vi "DecodeVireoToBotSpeak.vi"(3 "Via file":string="// Autogenerated Vireo assembly file\n// Generated on Fri Mar 27 10:48:11 2015\n\ndefine (c0 dv(.UInt32 1) )\ndefine (c1 dv(.UInt32 1) )\ndefine (c2 dv(c(\n    e(.String n0)   // Address\n    e(.String n1)   // Reply EOF\n    e(.String n2)   // Hardware\n    e(.Int8 n3)   // Retries\n    e(.Int32 n4)   // Timeout\n    e(.Boolean n5)   // Open?\n) ('' '' '' 0 0 false )) )\ndefine (c3 dv(.String '') )\n//---------------------------------------------------\n//VI Definition: BotSpeak_DIOWrite.vi\ndefine (videf1 dv(.VirtualInstrument (\n    c(\n        i(dv(.UInt32 1) local2)   // State\n        o(dv(.String '') local5)   // response\n        i(dv(c(\n            e(.String n0)   // Address\n            e(.String n1)   // Reply EOF\n            e(.String n2)   // Hardware\n            e(.Int8 n3)   // Retries\n            e(.Int32 n4)   // Timeout\n            e(.Boolean n5)   // Open?\n        ) ('' '' '' 0 0 false )) local1)   // Bot Settings\n        i(dv(.UInt32 0) local3)   // DIO Line\n        o(dv(c(\n            e(.String n0)   // Address\n            e(.String n1)   // Reply EOF\n            e(.String n2)   // Hardware\n            e(.Int8 n3)   // Retries\n            e(.Int32 n4)   // Timeout\n            e(.Boolean n5)   // Open?\n        ) ('' '' '' 0 0 false )) local4)   // Bot Settings\n    )\n    c(\n    )\n        clump(1\n        Copy(c2 local4 )\n        Copy(c3 local5 )\n//--- end of vi\n    )\n)))\n//---------------------------------------------------\n//VI Definition: TestingVI.vi\ndefine (videf2 dv(.VirtualInstrument (\n    c(\n    )\n        clump(1\n        videf1(c0 * * c1 *)\n//--- end of vi\n    )\n)))\nenqueue (videf2)\n") -> (1 "BotSpeak":string="SET DIO[1],1\n")   [LabVIEW 2012]
panel:
  out "params":T1(array[cluster])
  out "Array 3":string[](array[string])=["", "", "", "", "BotSpeak_DIOWrite.vi", "TestingVI.vi", ""]
  out "Array":T2(array[cluster])=[{"command"="define", "Contents"="c0 dv(.UInt32 1)", "previous comment"="// Generated on Fri Mar 27 10:48:11 2015"}, {"command"="define", "Contents"="c1 dv(.UInt32 1)", "previous comment"=""}, {"command"="define", "Contents"="c2 dv(c(\n    e(.String n0)   // Address\n    e(.String n1)   // Reply EOF\n    e(.String n2)   // Hardware\n    e(.Int8 n3)   // Retries\n    e(.Int32 n4)   // Timeout\n    e(.Boolean n5)   // Open?\n) ('' '' '' 0 0 false ))", "previous comment"=""}, {"command"="define", "Contents"="c3 dv(.String '')", "previous comment"=""}, {"command"="define", "Contents"="videf1 dv(.VirtualInstrument (\n    c(\n        i(dv(.UInt32 1) local2)   // State\n        o(dv(.String '') local5)   // response\n        i(dv(c(\n            e(.String n0)   // Address\n            e(.String n1)   // Reply EOF\n            e(.String n2)   // Hardware\n            e(.Int8 n3)   // Retries\n            e(.Int32 n4)   // Timeout\n            e(.Boolean n5)   // Open?\n        ) ('' '' '' 0 0 false )) local1)   // Bot Settings\n        i(dv(.UInt32 0) local3)   // DIO Line\n        o(dv(c(\n            e(.String n0)   // Address\n            e(.String n1)   // Reply EOF\n            e(.String n2)   // Hardware\n            e(.Int8 n3)   // Retries\n            e(.Int32 n4)   // Timeout\n            e(.Boolean n5)   // Open?\n        ) ('' '' '' 0 0 false )) local4)   // Bot Settings\n    )\n    c(\n    )\n        clump(1\n        Copy(c2 local4 )\n        Copy(c3 local5 )\n//--- end of vi\n    )\n))", "previous comment"="//VI Definition: BotSpeak_DIOWrite.vi"}, {"command"="define", "Contents"="videf2 dv(.VirtualInstrument (\n    c(\n    )\n        clump(1\n        videf1(c0 * * c1 *)\n//--- end of vi\n    )\n))", "previous comment"="//VI Definition: TestingVI.vi"}, {"command"="enqueue", "Contents"="videf2", "previous comment"=""}]
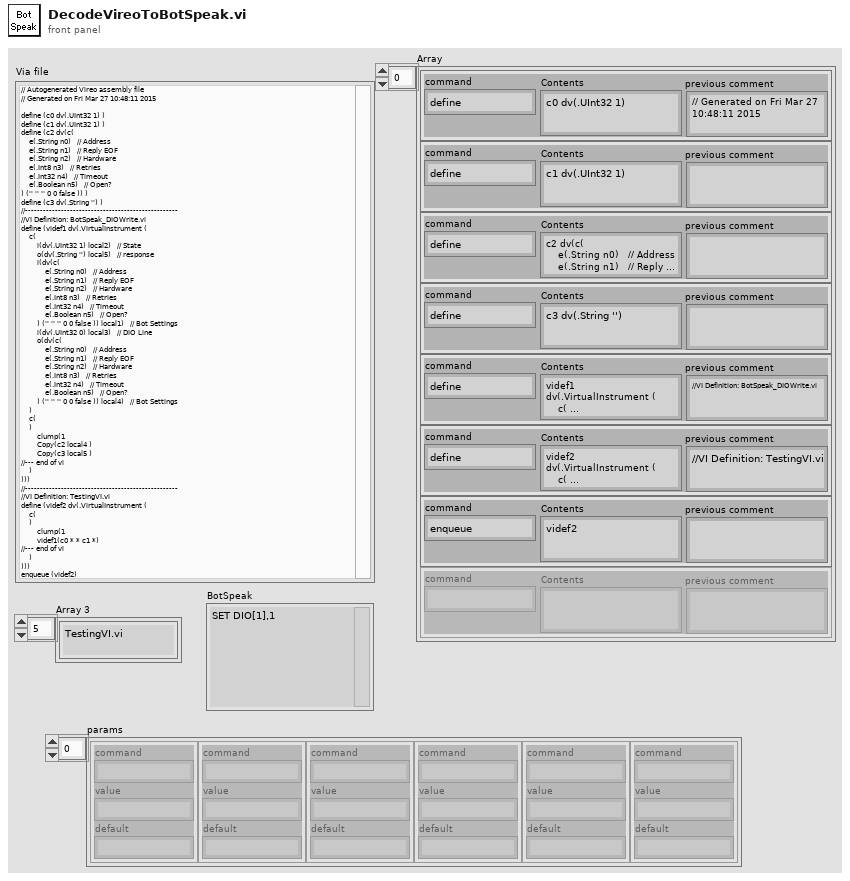
[diagram p1: front panel]
types:
  T1 = cluster{"command":string, "value":string, "default":string}[]
  T2 = cluster{"command":string, "Contents":string, "previous comment":string}[]
  T3 = cluster{"Contents":string, "Contents 2":string, "String":string}[]
  T4 = cluster{"command":string, "Contents":string, "Via file":string}
  T5 = cluster{"Contents":string, "String out":string, "defaults":string}
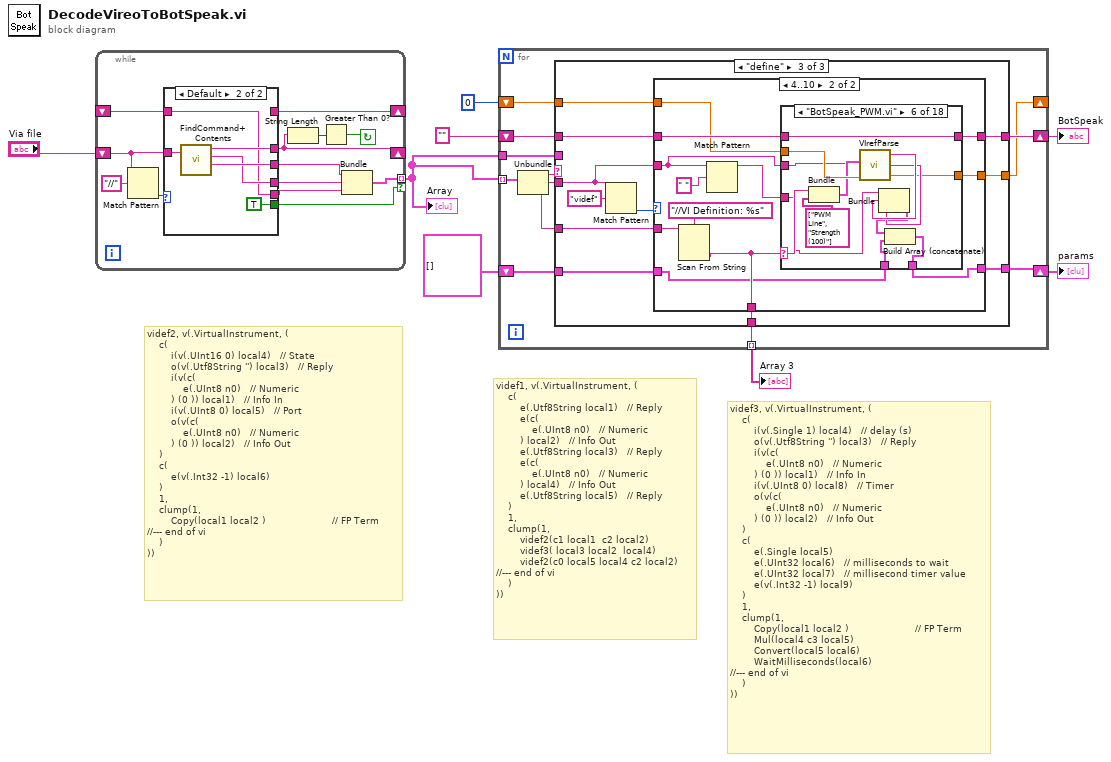
[diagram p0: block diagram]
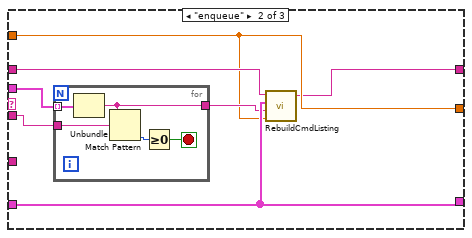
[diagram p3: hidden frame]
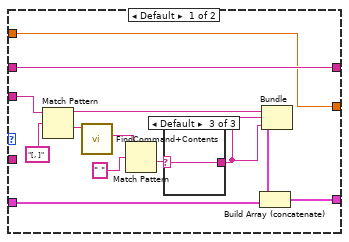
[diagram p4: hidden frame]
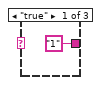
[diagram p5: hidden frame]
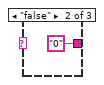
[diagram p6: hidden frame]
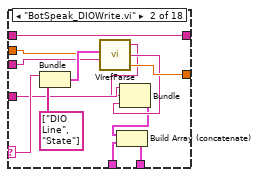
[diagram p8: hidden frame]
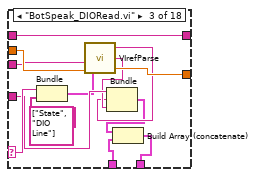
[diagram p9: hidden frame]
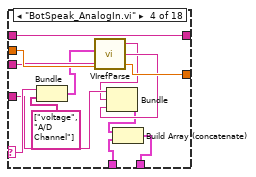
[diagram p10: hidden frame]
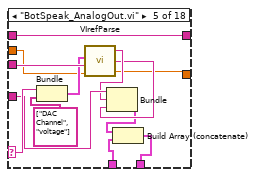
[diagram p11: hidden frame]
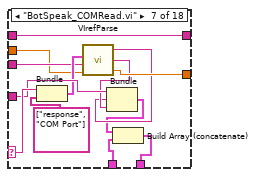
[diagram p12: hidden frame]
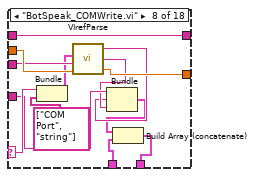
[diagram p13: hidden frame]
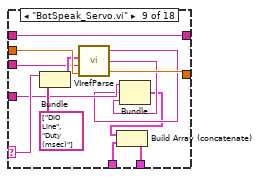
[diagram p14: hidden frame]
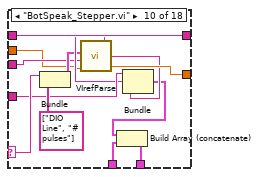
[diagram p15: hidden frame]
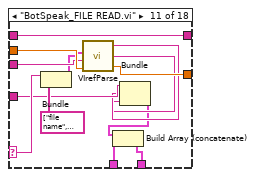
[diagram p16: hidden frame]
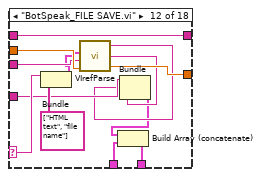
[diagram p17: hidden frame]
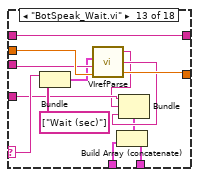
[diagram p18: hidden frame]
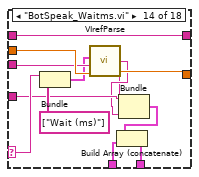
[diagram p19: hidden frame]
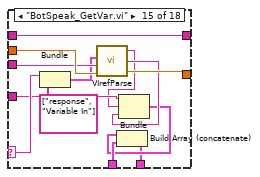
[diagram p20: hidden frame]
diagram:
  # "videf3, v(.VirtualInstrument, (\n    c(\n        i(v(.Single 1) local4)   // delay (s)\n        o(v(.Utf8String '') local3)   // Reply\n        i(v(c(\n            e(.UInt8 n0)   // Numeric\n        ) (0 )) local1)   // Info In\n        i(v(.UInt8 0) local8)   // Timer\n        o(v(c(\n            e(.UInt8 n0)   // Numeric\n        ) (0 )) local2)   // Info Out\n    )\n    c(\n        e(.Single local5)\n        e(.UInt32 local6)   // milliseconds to wait\n        e(.UInt32 local7)   // millisecond timer value\n        e(v(.Int32 -1) local9)\n    )\n    1,\n    clump(1,\n        Copy(local1 local2 )                      // FP Term\n        Mul(local4 c3 local5)\n        Convert(local5 local6)\n        WaitMilliseconds(local6)\n//--- end of vi\n    )\n))"
  # "videf1, v(.VirtualInstrument, (\n    c(\n        e(.Utf8String local1)   // Reply\n        e(c(\n            e(.UInt8 n0)   // Numeric\n        ) local2)   // Info Out\n        e(.Utf8String local3)   // Reply\n        e(c(\n            e(.UInt8 n0)   // Numeric\n        ) local4)   // Info Out\n        e(.Utf8String local5)   // Reply\n    )\n    1,\n    clump(1,\n        videf2(c1 local1  c2 local2)\n        videf3( local3 local2  local4)\n        videf2(c0 local5 local4 c2 local2)\n//--- end of vi\n    )\n))"
  # "videf2, v(.VirtualInstrument, (\n    c(\n        i(v(.UInt16 0) local4)   // State\n        o(v(.Utf8String '') local3)   // Reply\n        i(v(c(\n            e(.UInt8 n0)   // Numeric\n        ) (0 )) local1)   // Info In\n        i(v(.UInt8 0) local5)   // Port\n        o(v(c(\n            e(.UInt8 n0)   // Numeric\n        ) (0 )) local2)   // Info Out\n    )\n    c(\n        e(v(.Int32 -1) local6)\n    )\n    1,\n    clump(1,\n        Copy(local1 local2 )                      // FP Term\n//--- end of vi\n    )\n))"
  n1 = while {
    shift-right: [w21] -> _
    shift-left: "Via file" -> [w15]
    tunnel: [w16] -> w3 mode=indexing if=w10
    shift-right: [w12] -> _
    shift-left: _ -> [w11]
    stop <- w19 continue-if-true
    n2 = Match Pattern(string=w15, regular expression="//") -> (offset past match=w13:i32)  [unwired: 1 in, 3 out]
    n3 = case shown="Default" w13 {
      tunnel: [w24 w32] -> w21
      tunnel: ["//" ("regular expression") w31] -> w18
      tunnel: [w22 w30] -> w17
      tunnel: w15 -> [w26 w29]
      tunnel: [w22 _] -> w12
      tunnel: [_ w28] -> w9
      tunnel: w11 -> [_ w28]
      tunnel: [_ TRUE] -> w10
      frame 0..2 {
        n4 = Match Pattern(string=w26, regular expression="\n") -> (before substring=w22:string, after substring=w24:string)  [unwired: 1 in, 2 out]
      }
      frame Default {
        n5 = call <userlib>:"FindCommand+Contents.vi"("Via file in"=w29) -> ("left"=w32:string, "Contents"=w30:string, "command"=w31:string)  [unwired: 1 in, 1 out]
      }
    }
    n6 = String Length(string=w21) -> (length=w20:i32)
    n7 = Greater Than 0?(x=w20) -> (x > 0?=w19:bool)
    n8 = Bundle("command"=w18, "Contents"=w17, "Via file"=w9) -> (w16:T4)  [unwired: 1 in]
  }
  "Array" <- w3
  n9 = for {
    tunnel: w3 -> [w44] mode=indexing
    shift-right: [w39] -> w6
    shift-left: "" -> [w40]
    shift-right: [w33] -> w2
    shift-left: T3 [] ("Array") -> [w38]
    tunnel: [w37] -> w4 mode=indexing
    tunnel: w3 -> [w36]
    shift-right: [w34] -> _
    shift-left: 0 -> [w35]
    n10 = Unbundle(w44) -> ("command"=w43:string, "Contents"=w42:string, "Via file"=w41:string)
    n11 = case shown="\"define\"" w43 {
      tunnel: w42 -> [_ w53 w65]
      tunnel: w41 -> [_ _ w68]
      tunnel: w40 -> [w47 w52 w67]
      tunnel: [w47 w48 w66] -> w39
      tunnel: [w46 w51 w64] -> w33
      tunnel: w38 -> [w46 w51 w63]
      tunnel: [_ _ w62] -> w37
      tunnel: w36 -> [_ w54 _]
      tunnel: w35 -> [w45 w49 w61]
      tunnel: [w45 w49 w60] -> w34
      frame Default {
      }
      frame "enqueue" {
        n12 = for {
          tunnel: w54 -> [w59] mode=indexing
          tunnel: w53 -> [w58]
          tunnel: [w55] -> w50
          stop <- w56 stop-if-true
          n13 = Unbundle(w59) -> ("Contents"=w55:string)  [unwired: 2 out]
          n14 = Match Pattern(string=w55, regular expression=w58) -> (offset past match=w57:i32)  [unwired: 1 in, 3 out]
          n15 = Greater Or Equal To 0?(x=w57) -> (x >= 0?=w56:bool)
        }
        n16 = call <userlib>:"RebuildCmdListing.vi"("Numeric"=w49, "Contents"=w50, "Params"=w51, "String in"=w52) -> ("String out"=w48:string)  [unwired: 1 in, 1 out]
      }
      frame "define" {
        n17 = Match Pattern(string=w65, regular expression="videf") -> (offset past match=w69:i32)  [unwired: 1 in, 3 out]
        n18 = case shown="4..10" w69 {
          tunnel: w68 -> [_ w98]
          tunnel: w67 -> [w83 w96]
          tunnel: [w83 w95] -> w66
          tunnel: w65 -> [w81 w93]
          tunnel: [w71 w89] -> w64
          tunnel: w63 -> [w75 w90]
          tunnel: [_ w94] -> w62
          tunnel: w61 -> [w72 w88]
          tunnel: [w72 w87] -> w60
          frame Default {
            n19 = Match Pattern(string=w81, regular expression="[, ]") -> (before substring=w79:string, after substring=w80:string)  [unwired: 1 in, 2 out]
            n20 = call <userlib>:"FindCommand+Contents.vi"("Via file in"=w80) -> ("Contents"=w78:string)  [unwired: 1 in, 3 out]
            n21 = Match Pattern(string=w78, regular expression=" ") -> (after substring=w74:string)  [unwired: 1 in, 3 out]
            n22 = case shown="Default" w74 {
              selector: w74 -> [_ _ w86]
              tunnel: ["1" "0" w86] -> w73
              frame "true" {
              }
              frame "false" {
              }
              frame Default {
              }
            }
            n23 = Bundle("Contents"=w79, w73, w73) -> (w76:cluster{"Contents":string, string, string})  [unwired: 1 in]
            n24 = Build Array (concatenate)(w76, w75) -> (w71:T3)
          }
          frame 4..10 {
            n25 = Scan From String(format string="//VI Definition: %s" ("regular expression"), input string=w98) -> (output 1=w94:string)  [unwired: 3 in, 3 out]
            n26 = Match Pattern(string=w93, regular expression=" ") -> (before substring=w91:string)  [unwired: 1 in, 3 out]
            n27 = case shown="\"BotSpeak_PWM.vi\"" w94 {
              selector: w94 -> [_ w114 w126 w139 w152 w165 w178 w191 w205 w218 w231 w244 w257 w270 w283 w296 w309 w322]
              tunnel: w96 -> [w101 w112 w127 w140 w153 w166 w179 w192 w203 w216 w229 w242 w255 w268 w281 w294 w307 w320]
              tunnel: [w101 w112 w127 w140 w153 w166 w179 w192 w203 w216 w229 w242 w255 w268 w281 w294 w307 w320] -> w95
              tunnel: w93 -> [_ w108 w120 w134 w148 w159 w173 w186 w197 w208 w224 w237 w251 w263 w276 w288 w302 w313]
              tunnel: w91 -> [_ w111 w125 w137 w151 w164 w177 w190 w202 w215 w228 w241 w254 w267 w280 w293 w306 w319]
              tunnel: w90 -> [w100 w110 w124 w136 w150 w163 w176 w189 w201 w214 w227 w240 w253 w266 w279 w292 w305 w318]
              tunnel: [w100 w102 w115 w128 w141 w154 w167 w180 w193 w213 w220 w232 w245 w258 w271 w291 w297 w310] -> w89
              tunnel: w88 -> [w99 w107 w122 w135 w142 w161 w172 w187 w200 w207 w225 w239 w252 w265 w278 w290 w304 w317]
              tunnel: [w99 w106 w121 w132 w143 w156 w171 w184 w199 w212 w226 w238 w249 w264 w277 w289 w303 w316] -> w87
              frame Default {
              }
              frame "BotSpeak_DIOWrite.vi" {
                n28 = Bundle(w114, string[] ["DIO Line", "State"]) -> (w109:cluster{string, string[]})  [unwired: 1 in]
                n29 = call <userlib>:"VIrefParse.vi"("Var Number"=w107, "VIA"=w108, "Params"=w109) -> ("Var Number 2"=w106:dbl, "defaults"=w105:string, "String out"=w104:string)  [unwired: 1 in]
                n30 = Bundle("Contents"=w111, "String out"=w104, "defaults"=w105) -> (w103:T5)  [unwired: 1 in]
                n31 = Build Array (concatenate)(w103, w110) -> (w102:T3)
              }
              frame "BotSpeak_DIORead.vi" {
                n32 = Bundle(w126, string[] ["State", "DIO Line"]) -> (w119:cluster{string, string[]})  [unwired: 1 in]
                n33 = call <userlib>:"VIrefParse.vi"("Var Number"=w122, "VIA"=w120, "Params"=w119) -> ("Var Number 2"=w121:dbl, "defaults"=w118:string, "String out"=w117:string)  [unwired: 1 in]
                n34 = Bundle("Contents"=w125, "String out"=w117, "defaults"=w118) -> (w116:T5)  [unwired: 1 in]
                n35 = Build Array (concatenate)(w116, w124) -> (w115:T3)
              }
              frame "BotSpeak_AnalogIn.vi" {
                n36 = Bundle(w139, string[] ["voltage", "A/D Channel"]) -> (w133:cluster{string, string[]})  [unwired: 1 in]
                n37 = call <userlib>:"VIrefParse.vi"("Var Number"=w135, "VIA"=w134, "Params"=w133) -> ("Var Number 2"=w132:dbl, "defaults"=w131:string, "String out"=w130:string)  [unwired: 1 in]
                n38 = Bundle("Contents"=w137, "String out"=w130, "defaults"=w131) -> (w129:T5)  [unwired: 1 in]
                n39 = Build Array (concatenate)(w129, w136) -> (w128:T3)
              }
              frame "BotSpeak_AnalogOut.vi" {
                n40 = Bundle(w152, string[] ["DAC Channel", "voltage"]) -> (w147:cluster{string, string[]})  [unwired: 1 in]
                n41 = call <userlib>:"VIrefParse.vi"("Var Number"=w142, "VIA"=w148, "Params"=w147) -> ("Var Number 2"=w143:dbl, "defaults"=w145:string, "String out"=w146:string)  [unwired: 1 in]
                n42 = Bundle("Contents"=w151, "String out"=w146, "defaults"=w145) -> (w144:T5)  [unwired: 1 in]
                n43 = Build Array (concatenate)(w144, w150) -> (w141:T3)
              }
              frame "BotSpeak_PWM.vi" {
                n44 = Bundle(w165, string[] ["PWM Line", "Strength (100)"]) -> (w160:cluster{string, string[]})  [unwired: 1 in]
                n45 = call <userlib>:"VIrefParse.vi"("Var Number"=w161, "Params"=w160, "String in"=w159) -> ("Var Number 2"=w156:dbl, "defaults"=w157:string, "String out"=w158:string)  [unwired: 1 in]
                n46 = Bundle("Contents"=w164, "String out"=w158, "defaults"=w157) -> (w155:T5)  [unwired: 1 in]
                n47 = Build Array (concatenate)(w155, w163) -> (w154:T3)
              }
              frame "BotSpeak_COMRead.vi" {
                n48 = Bundle(w178, string[] ["response", "COM Port"]) -> (w174:cluster{string, string[]})  [unwired: 1 in]
                n49 = call <userlib>:"VIrefParse.vi"("Var Number"=w172, "VIA"=w173, "Params"=w174) -> ("Var Number 2"=w171:dbl, "defaults"=w170:string, "String out"=w169:string)  [unwired: 1 in]
                n50 = Bundle("Contents"=w177, "String out"=w169, "defaults"=w170) -> (w168:T5)  [unwired: 1 in]
                n51 = Build Array (concatenate)(w168, w176) -> (w167:T3)
              }
              frame "BotSpeak_COMWrite.vi" {
                n52 = Bundle(w191, string[] ["COM Port", "string"]) -> (w185:cluster{string, string[]})  [unwired: 1 in]
                n53 = call <userlib>:"VIrefParse.vi"("Var Number"=w187, "VIA"=w186, "Params"=w185) -> ("Var Number 2"=w184:dbl, "defaults"=w183:string, "String out"=w182:string)  [unwired: 1 in]
                n54 = Bundle("Contents"=w190, "String out"=w182, "defaults"=w183) -> (w181:T5)  [unwired: 1 in]
                n55 = Build Array (concatenate)(w181, w189) -> (w180:T3)
              }
              frame "BotSpeak_Servo.vi" {
                n56 = Bundle(w205, string[] ["DIO Line", "Duty (msec)"]) -> (w198:cluster{string, string[]})  [unwired: 1 in]
                n57 = call <userlib>:"VIrefParse.vi"("Var Number"=w200, "VIA"=w197, "Params"=w198) -> ("Var Number 2"=w199:dbl, "defaults"=w196:string, "String out"=w195:string)  [unwired: 1 in]
                n58 = Bundle("Contents"=w202, "String out"=w195, "defaults"=w196) -> (w194:T5)  [unwired: 1 in]
                n59 = Build Array (concatenate)(w194, w201) -> (w193:T3)
              }
              frame "BotSpeak_Stepper.vi" {
                n60 = Bundle(w218, string[] ["DIO Line", "# pulses"]) -> (w209:cluster{string, string[]})  [unwired: 1 in]
                n61 = call <userlib>:"VIrefParse.vi"("Var Number"=w207, "VIA"=w208, "Params"=w209) -> ("Var Number 2"=w212:dbl, "defaults"=w211:string, "String out"=w210:string)  [unwired: 1 in]
                n62 = Bundle("Contents"=w215, "String out"=w210, "defaults"=w211) -> (w206:T5)  [unwired: 1 in]
                n63 = Build Array (concatenate)(w206, w214) -> (w213:T3)
              }
              frame "BotSpeak_FILE READ.vi" {
                n64 = Bundle(w231, string[] ["file name", "DIO Line"]) -> (w223:cluster{string, string[]})  [unwired: 1 in]
                n65 = call <userlib>:"VIrefParse.vi"("Var Number"=w225, "VIA"=w224, "Params"=w223) -> ("Var Number 2"=w226:dbl, "defaults"=w221:string, "String out"=w222:string)  [unwired: 1 in]
                n66 = Bundle("Contents"=w228, "String out"=w222, "defaults"=w221) -> (w219:T5)  [unwired: 1 in]
                n67 = Build Array (concatenate)(w219, w227) -> (w220:T3)
              }
              frame "BotSpeak_FILE SAVE.vi" {
                n68 = Bundle(w244, string[] ["HTML text", "file name"]) -> (w236:cluster{string, string[]})  [unwired: 1 in]
                n69 = call <userlib>:"VIrefParse.vi"("Var Number"=w239, "VIA"=w237, "Params"=w236) -> ("Var Number 2"=w238:dbl, "defaults"=w235:string, "String out"=w234:string)  [unwired: 1 in]
                n70 = Bundle("Contents"=w241, "String out"=w234, "defaults"=w235) -> (w233:T5)  [unwired: 1 in]
                n71 = Build Array (concatenate)(w233, w240) -> (w232:T3)
              }
              frame "BotSpeak_Wait.vi" {
                n72 = Bundle(w257, string[] ["Wait (sec)"]) -> (w250:cluster{string, string[]})  [unwired: 1 in]
                n73 = call <userlib>:"VIrefParse.vi"("Var Number"=w252, "VIA"=w251, "Params"=w250) -> ("Var Number 2"=w249:dbl, "defaults"=w248:string, "String out"=w247:string)  [unwired: 1 in]
                n74 = Bundle("Contents"=w254, "String out"=w247, "defaults"=w248) -> (w246:T5)  [unwired: 1 in]
                n75 = Build Array (concatenate)(w246, w253) -> (w245:T3)
              }
              frame "BotSpeak_Waitms.vi" {
                n76 = Bundle(w270, string[] ["Wait (ms)"]) -> (w262:cluster{string, string[]})  [unwired: 1 in]
                n77 = call <userlib>:"VIrefParse.vi"("Var Number"=w265, "VIA"=w263, "Params"=w262) -> ("Var Number 2"=w264:dbl, "defaults"=w261:string, "String out"=w260:string)  [unwired: 1 in]
                n78 = Bundle("Contents"=w267, "String out"=w260, "defaults"=w261) -> (w259:T5)  [unwired: 1 in]
                n79 = Build Array (concatenate)(w259, w266) -> (w258:T3)
              }
              frame "BotSpeak_GetVar.vi" {
                n80 = Bundle(w283, string[] ["response", "Variable In"]) -> (w275:cluster{string, string[]})  [unwired: 1 in]
                n81 = call <userlib>:"VIrefParse.vi"("Var Number"=w278, "VIA"=w276, "Params"=w275) -> ("Var Number 2"=w277:dbl, "defaults"=w274:string, "String out"=w273:string)  [unwired: 1 in]
                n82 = Bundle("Contents"=w280, "String out"=w273, "defaults"=w274) -> (w272:T5)  [unwired: 1 in]
                n83 = Build Array (concatenate)(w272, w279) -> (w271:T3)
              }
              frame "BotSpeak_Set.vi" {
                n84 = Bundle(w296, string[] ["Variable In", "value"]) -> (w287:cluster{string, string[]})  [unwired: 1 in]
                n85 = call <userlib>:"VIrefParse.vi"("Var Number"=w290, "VIA"=w288, "Params"=w287) -> ("Var Number 2"=w289:dbl, "defaults"=w286:string, "String out"=w285:string)  [unwired: 1 in]
                n86 = Bundle("Contents"=w293, "String out"=w285, "defaults"=w286) -> (w284:T5)  [unwired: 1 in]
                n87 = Build Array (concatenate)(w284, w292) -> (w291:T3)
              }
              frame "BotSpeak_GetVer.vi" {
                n88 = Bundle(w309, string[] ["version"]) -> (w301:cluster{string, string[]})  [unwired: 1 in]
                n89 = call <userlib>:"VIrefParse.vi"("Var Number"=w304, "VIA"=w302, "Params"=w301) -> ("Var Number 2"=w303:dbl, "defaults"=w300:string, "String out"=w299:string)  [unwired: 1 in]
                n90 = Bundle("Contents"=w306, "String out"=w299, "defaults"=w300) -> (w298:T5)  [unwired: 1 in]
                n91 = Build Array (concatenate)(w298, w305) -> (w297:T3)
              }
              frame "BotSpeak_System.vi" {
                n92 = Bundle(w322, string[] ["Variable In", "Values sent"]) -> (w312:cluster{string, string[]})  [unwired: 1 in]
                n93 = call <userlib>:"VIrefParse.vi"("Var Number"=w317, "VIA"=w313, "Params"=w312) -> ("Var Number 2"=w316:dbl, "defaults"=w315:string, "String out"=w314:string)  [unwired: 1 in]
                n94 = Bundle("Contents"=w319, "String out"=w314, "defaults"=w315) -> (w311:T5)  [unwired: 1 in]
                n95 = Build Array (concatenate)(w311, w318) -> (w310:T3)
              }
            }
          }
        }
      }
    }
  }
  "BotSpeak" <- w6
  "Array 3" <- w4
  "params" <- w2
